vi "Get Measurement Details.vi"(8 "error in":errorcluster) -> (0 "error out":errorcluster, 1 "Measurement Annotations":T1[](array[typedef]), 2 "Service Class":string, 3 "Measurement Details":T2)   [LabVIEW 2020, in "NIDigitalSPI.lvlib"]
uses:
  NIDigitalSPI.lvlib
  <vilib>/MeasurementLink/MeasurementLink Measurement Server Internal/RPC Messages/ni_measurementlink_measurement_v1_MeasurementDetails.ctl
  <vilib>/MeasurementLink/MeasurementLink Measurement Server/Helpers/TypeDefs/Measurement Annotation.ctl
  <vilib>/MeasurementLink/MeasurementLink Measurement Server Internal/MeasurementLink Measurement Server Internal.lvlib
  <vilib>/MeasurementLink/MeasurementLink Measurement Server/MeasurementLink Measurement Server.lvlib
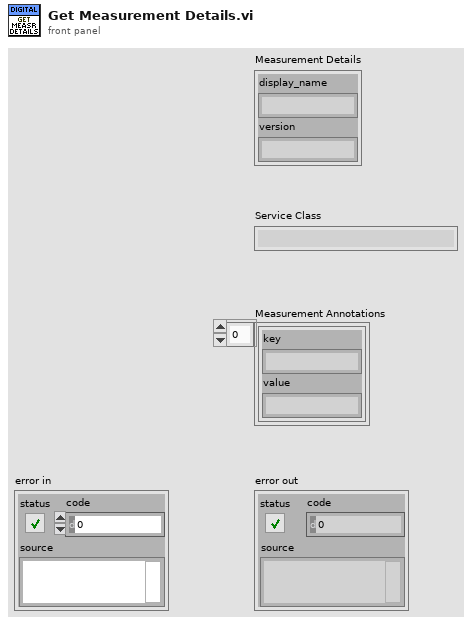
[diagram p1: front panel]
types:
  T1 = typedef "MeasurementLink Measurement Server.lvlib/Measurement Annotation.ctl" = cluster{"key":string, "value":string}
  T2 = typedef "MeasurementLink Measurement Server Internal.lvlib/ni_measurementlink_measurement_v1_MeasurementDetails.ctl" = cluster{"display_name":string, "version":string}
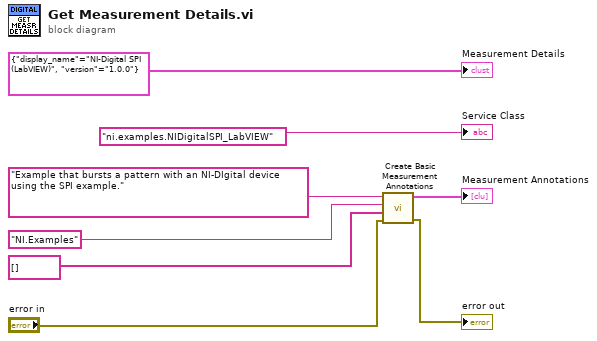
[diagram p0: block diagram]
diagram:
  n1 = call <vilib>:"Create Basic Measurement Annotations.vi"("error in"="error in", "Tags"=string[] [] ("ni/service.tags"), "Collection"="NI.Examples" ("ni/service.collection"), "Description"="Example that bursts a pattern with an NI-DIgital device using the SPI example." ("ni/service.description")) -> ("error out"=→"error out":errorcluster, "Measurement Annotations"=→"Measurement Annotations":T1[])  [unwired: 6 in]
  "Measurement Details" <- T2 {"display_name"="NI-Digital SPI (LabVIEW)", "version"="1.0.0"} ("Measurement Details")
  "Service Class" <- "ni.examples.NIDigitalSPI_LabVIEW" ("Service Class")
